vi "WCA_GET_CLNA.vi"(0 "Cartridge Band":u32=10, 1 "Slave Node in":cluster{"Address":i16, "Serial Number":i8[]}={"Address"=19, "Serial Number"=[16, 71, 55, 76, 1, 8, 0, -15]} {"Serial Number" format="%.0x"; "Address" format="%.0x"}, 2 "ObjHandle in":u32, 5 "POL":u32, 7 "sb":u32=1, 9 "avg":u32=1, 11 "error in (no error)":errorcluster) -> (4 "ObjHandle out":u32=92930112, 8 "CLNA_monitor":T1 {"Pol0 LNA1 S3 Gate V [V]" format="%.2f"; "Pol0 LNA1 S3 Drain C [mA]" format="%.2f"; "Pol0 LNA1 S3 Drain V [V]" format="%.2f"; "Pol0 LNA1 S2 Gate V [V]" format="%.2f"; "Pol0 LNA1 S2 Drain C [mA]" format="%.2f"; "Pol0 LNA1 S2 Drain V [V]" format="%.2f"; "Pol0 LNA1 S1 Gate V [V]" format="%.2f"; "Pol0 LNA1 S1 Drain C [mA]" format="%.2f"; "Pol0 LNA1 S1 Drain V [V]" format="%.2f"}, 15 "error out":errorcluster)   [LabVIEW 2017]
uses:
  WCA_Global.vi
  <vilib>/express/express arith-compare/Formula/XNode/ExpressFormulaBlockNode.xnode
panel:
  # "CLNA State."
  # "Vd [V]"
  # "Id [mA]"
  # "Vg [V]"
  # "Stage 1"
  # "Stage 2"
  # "Stage 3"
  # "Node Address"
  # "Serial Number"
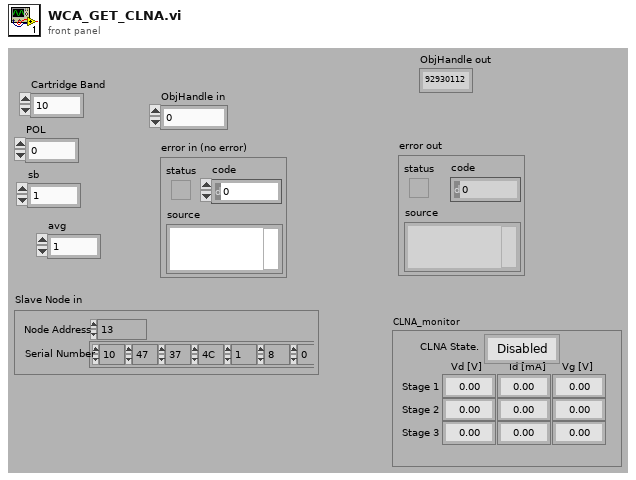
[diagram p1: front panel]
types:
  T1 = cluster{"Pol0 LNA1 S1 Drain V [V]":sgl, "Pol0 LNA1 S1 Drain C [mA]":sgl, "Pol0 LNA1 S1 Gate V [V]":sgl, "Pol0 LNA1 S2 Drain V [V]":sgl, "Pol0 LNA1 S2 Drain C [mA]":sgl, "Pol0 LNA1 S2 Gate V [V]":sgl, "Pol0 LNA1 S3 Drain V [V]":sgl, "Pol0 LNA1 S3 Drain C [mA]":sgl, "Pol0 LNA1 S3 Gate V [V]":sgl, "Pol0 LNA1 State":enum16{"Disabled", "Enabled"}}
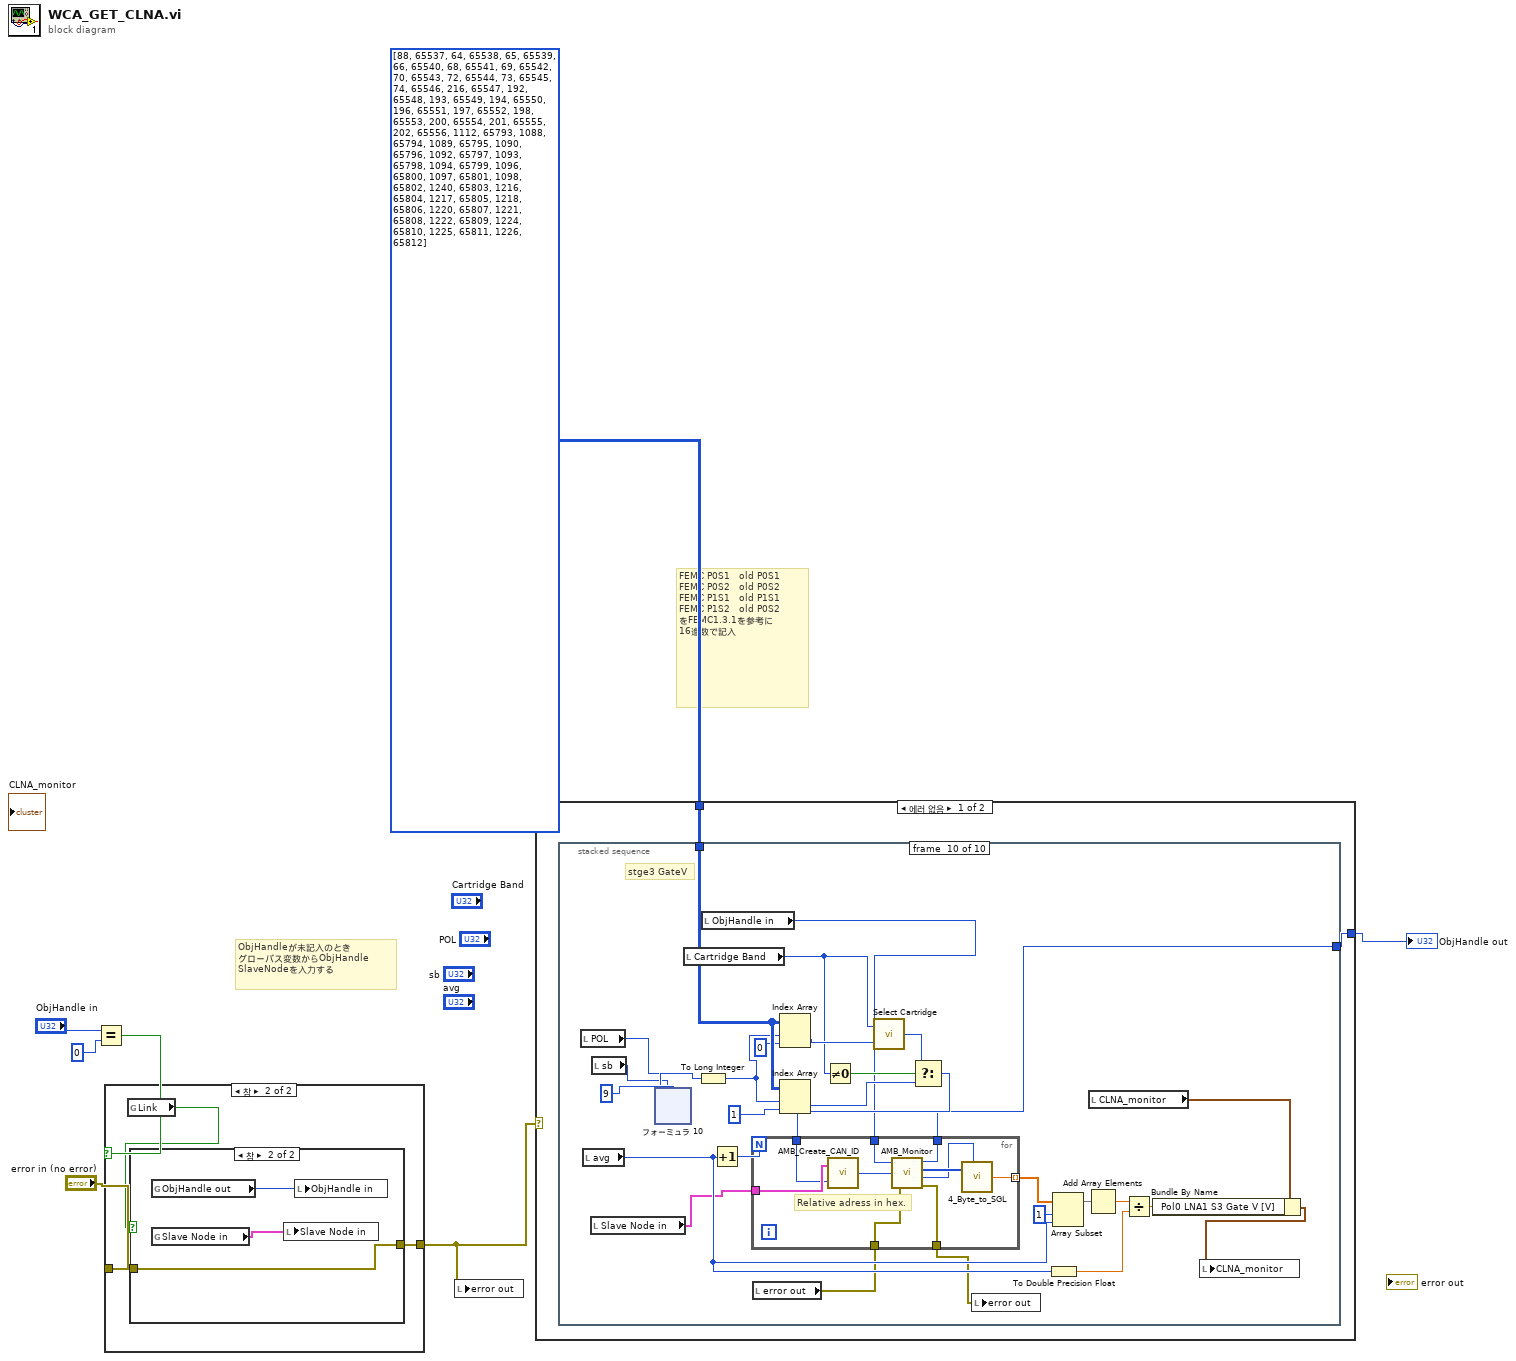
[diagram p0: block diagram]
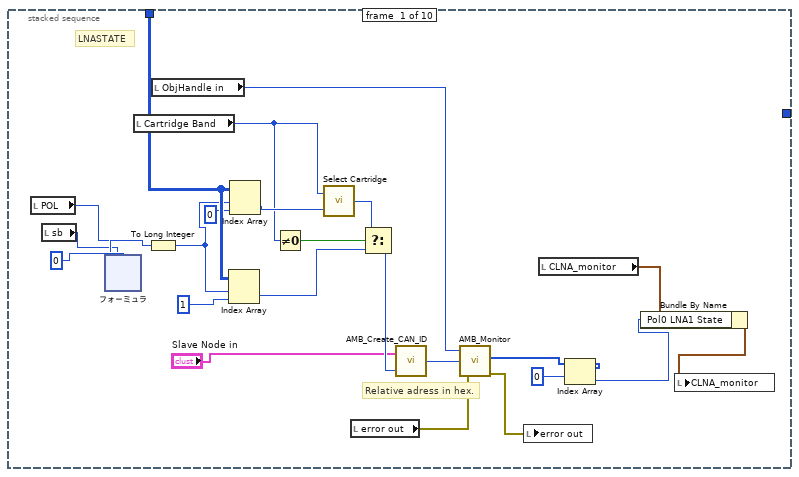
[diagram p2: hidden frame]
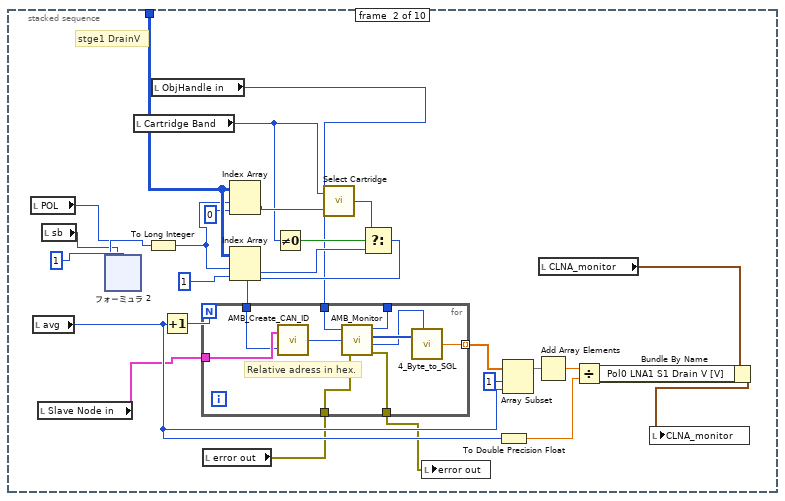
[diagram p3: hidden frame]
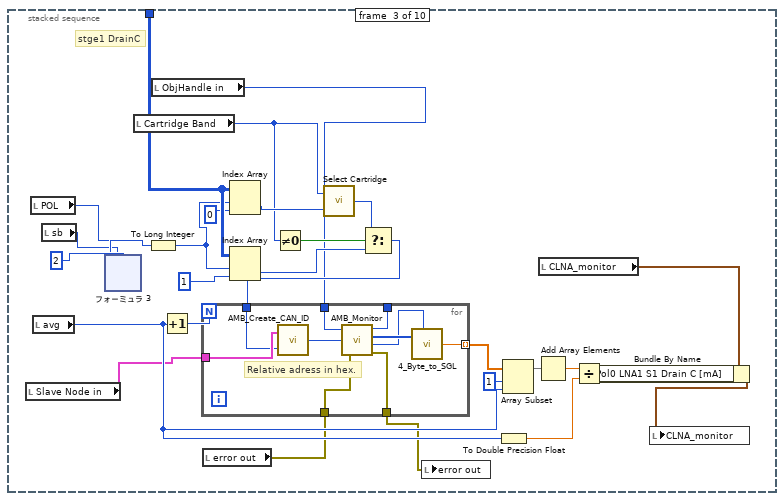
[diagram p4: hidden frame]
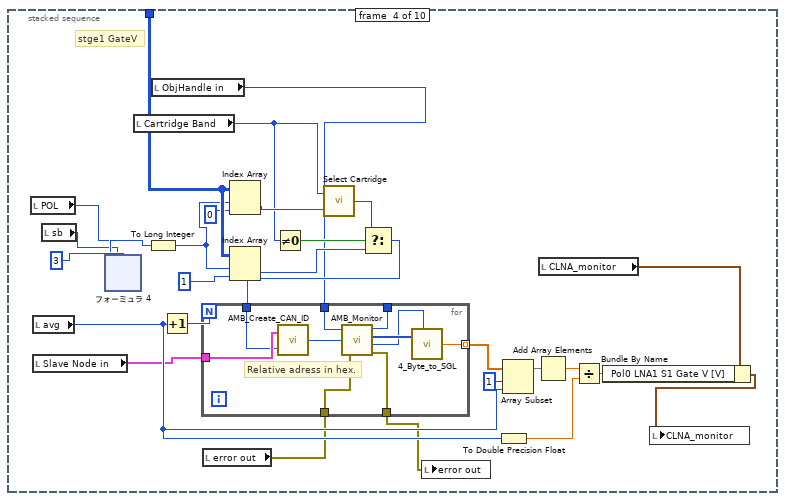
[diagram p5: hidden frame]
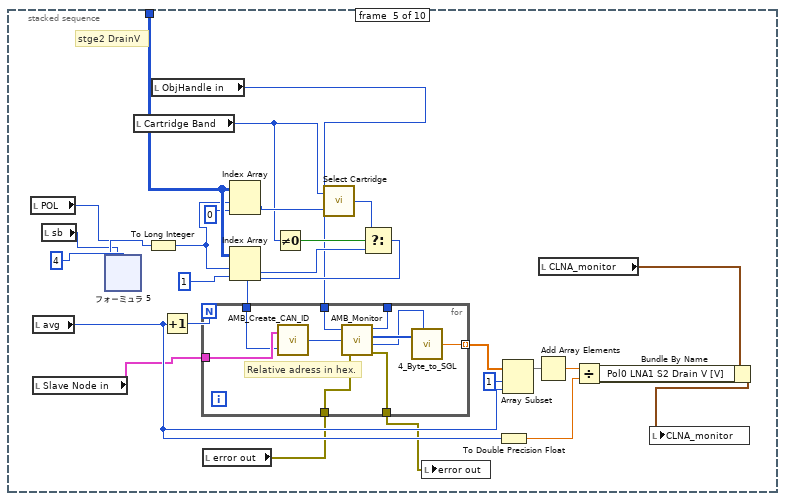
[diagram p6: hidden frame]
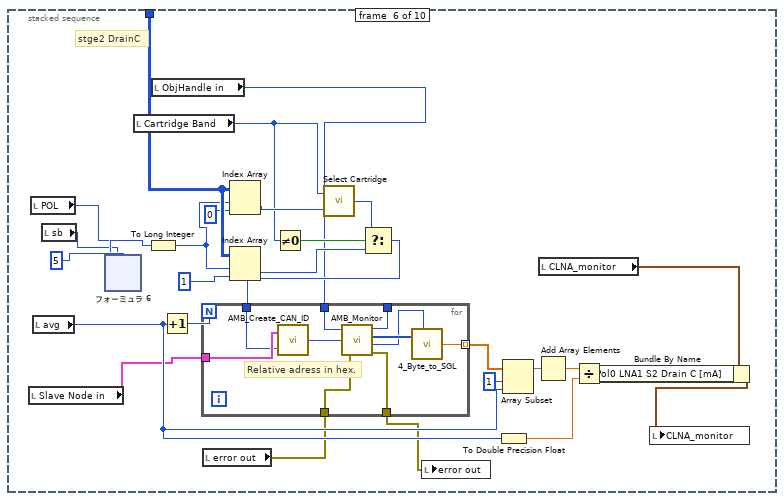
[diagram p7: hidden frame]
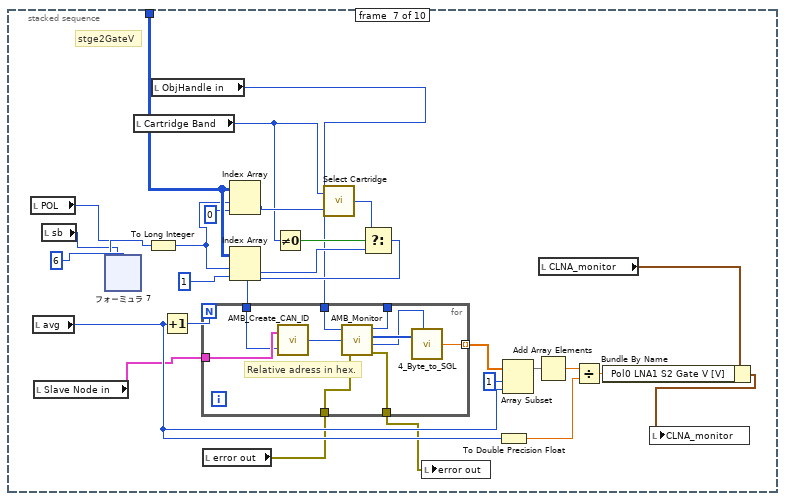
[diagram p8: hidden frame]
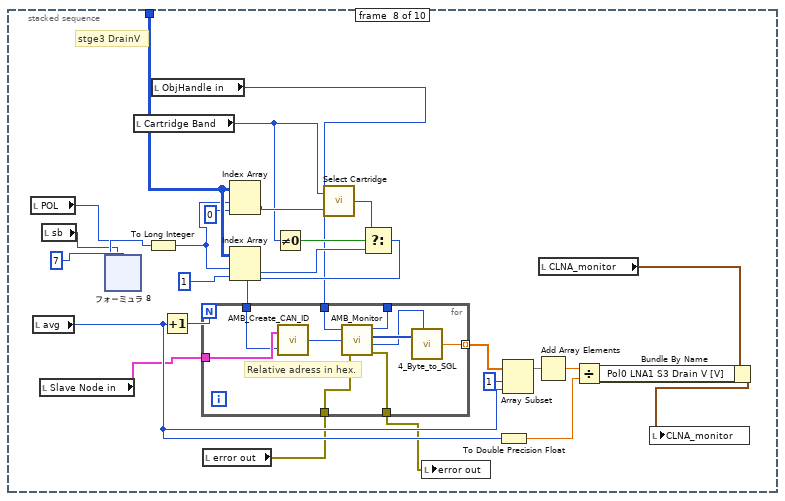
[diagram p9: hidden frame]
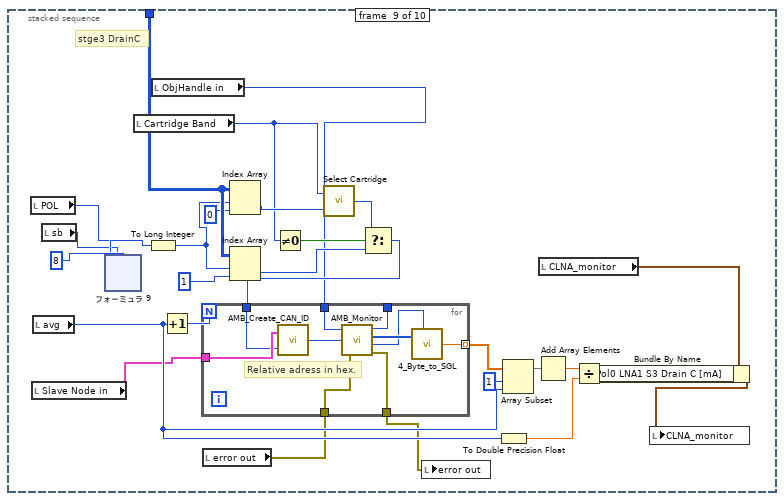
[diagram p10: hidden frame]
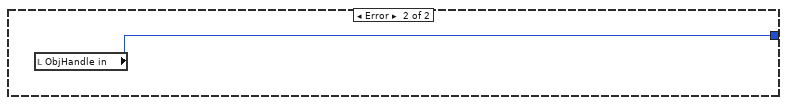
[diagram p11: hidden frame]
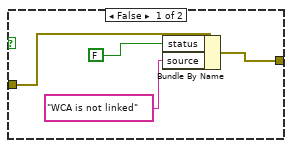
[diagram p13: hidden frame]
diagram:
  # "ObjHandleが未記入のとき\nグローバス変数からObjHandle\nSlaveNodeを入力する"
  # "FEMC P0S1   old P0S1\nFEMC P0S2   old P0S2\nFEMC P1S1   old P1S1\nFEMC P1S2   old P0S2\nをFEMC1.3.1を参考に\n16進数で記入"
  n1 = Equal?(x="ObjHandle in", y=0) -> (x = y?=w5:bool)
  n2 = case shown="참" w5 {
    tunnel: "error in (no error)" -> [w8 w11]
    tunnel: [w8 w10] -> w2
    frame False {
    }
    frame True {
      n3 = global read "WCA_Global.vi" "Link"() -> (w9:bool)
      n4 = case shown="참" w9 {
        tunnel: w11 -> [w15 w16]
        tunnel: [w12 w16] -> w10
        frame False {
          n5 = Bundle By Name(cluster=w15, "status"=FALSE, "source"="WCA is not linked") -> (w12:errorcluster)
        }
        frame True {
          n6 = global read "WCA_Global.vi" "ObjHandle out"() -> (w18:u32)
          n7 = global read "WCA_Global.vi" "Slave Node in"() -> (w17:cluster{"Address":i16, "Serial Number":i8[]})
          n8 = local write "Slave Node in"(w17) -> ()
          n9 = local write "ObjHandle in"(w18) -> ()
        }
      }
    }
  }
  n10 = local write "error out"(w2) -> ()
  n11 = case shown="에러 없음" w2 {
    tunnel: [w19 w508] -> w1
    tunnel: i32[][] [[88, 65537], [64, 65538], [65, 65539], [66, 65540], [68, 65541], [69, 65542], [70, 65543], [72, 65544], [73, 65545], [74, 65546], [216, 65547], [192, 65548], [193, 65549], [194, 65550], [196, 65551], [197, 65552], [198, 65553], [200, 65554], [201, 65555], [202, 65556], [1112, 65793], [1088, 65794], [1089, 65795], [1090, 65796], [1092, 65797], [1093, 65798], [1094, 65799], [1096, 65800], [1097, 65801], [1098, 65802], [1240, 65803], [1216, 65804], [1217, 65805], [1218, 65806], [1220, 65807], [1221, 65808], [1222, 65809], [1224, 65810], [1225, 65811], [1226, 65812]] -> [w20 _]
    frame No Error {
      n12 = stacked-sequence {
        tunnel: w20 -> [w44 w84 w134 w184 w234 w284 w334 w384 w434 w485]
        tunnel: [_ _ _ _ _ _ _ _ _ w457] -> w19
        frame #0 {
          # "Relative adress in hex."
          # "LNASTATE"
          n13 = local read "POL"() -> (w22:u32)
          n14 = local read "sb"() -> (w21:u32)
          n15 = xnode "フォーミュラ"("Pol"=w22, "sb"=w21, "n"=0) -> ("結果"=w33:u32)  [unwired: 1 in, 1 out]
          n16 = local read "Cartridge Band"() -> (w23:u32)
          n17 = To Long Integer(number=w33) -> (32bit integer=w32:i32)
          n18 = local read "ObjHandle in"() -> (w39:u32)
          n19 = Index Array(array=w44, index (row)=w32, index (col)=1) -> (element=w38:i32)
          n20 = Index Array(array=w44, index (row)=w32, index (col)=0) -> (element=w37:i32)
          n21 = Not Equal To 0?(x=w23) -> (x != 0?=w41:bool)
          n22 = call "Select Cartridge.vi"("Relative Address in"=w37, "Cartridge band"=w23) -> ("Relative Address out"=w42:u32)
          n23 = local read "error out"() -> (w25:errorcluster)
          n24 = Select(t=w42, s=w41, f=w38) -> (s? t:f=w43:u32)
          n25 = call "AMB_Create_CAN_ID.vi"("Relative Address in"=w43, "Slave Node in"="Slave Node in") -> ("CAN ID out"=w31:u32)
          n26 = call "AMB_Monitor.vi"("ObjHandle in"=w39, "CAN ID in"=w31, "error in"=w25) -> ("Data Array out"=w30:u8[], "error out"=w24:errorcluster)  [unwired: 2 out]
          n27 = local write "error out"(w24) -> ()
          n28 = local read "CLNA_monitor"() -> (w28:T1)
          n29 = Index Array(array=w30, index=0) -> (element=w27:u8)
          n30 = Bundle By Name(cluster=w28, "Pol0 LNA1 State"=w27) -> (w26:T1)
          n31 = local write "CLNA_monitor"(w26) -> ()
        }
        frame #1 {
          # "stge1 DrainV"
          n32 = local read "POL"() -> (w71:u32)
          n33 = local read "avg"() -> (w63:u32)
          n34 = local read "Slave Node in"() -> (w57:cluster{"Address":i16, "Serial Number":i8[]})
          n35 = local read "sb"() -> (w70:u32)
          n36 = xnode "フォーミュラ 2"("Pol"=w71, "sb"=w70, "n"=1) -> ("結果"=w76:u32)  [unwired: 1 in, 1 out]
          n37 = local read "Cartridge Band"() -> (w72:u32)
          n38 = To Long Integer(number=w76) -> (32bit integer=w75:i32)
          n39 = local read "ObjHandle in"() -> (w61:u32)
          n40 = Increment(x=w63) -> (x+1=w65:u32)
          n41 = local read "error out"() -> (w59:errorcluster)
          n42 = Index Array(array=w84, index (row)=w75, index (col)=0) -> (element=w80:i32)
          n43 = Index Array(array=w84, index (row)=w75, index (col)=1) -> (element=w81:i32)
          n44 = Not Equal To 0?(x=w72) -> (x != 0?=w82:bool)
          n45 = call "Select Cartridge.vi"("Relative Address in"=w80, "Cartridge band"=w72) -> ("Relative Address out"=w83:u32)
          n46 = Select(t=w83, s=w82, f=w81) -> (s? t:f=w62:u32)
          n47 = for {
            N: w65 -> [_]
            tunnel: [w105] -> _
            tunnel: [w104] -> w58
            tunnel: [w102] -> w66 mode=indexing
            tunnel: w57 -> [w100]
            tunnel: w62 -> [w99]
            tunnel: w61 -> [w98]
            tunnel: w59 -> [w97]
            # "Relative adress in hex."
            n48 = call "AMB_Create_CAN_ID.vi"("Relative Address in"=w99, "Slave Node in"=w100) -> ("CAN ID out"=w106:u32)
            n49 = call "AMB_Monitor.vi"("ObjHandle in"=w98, "CAN ID in"=w106, "error in"=w97) -> ("ObjHandle out"=w105:u32, "Data Array out"=w103:u8[], "Data Length out"=w101:u8, "error out"=w104:errorcluster)
            n50 = call "4_Byte_to_SGL.vi"("Array of 4 bytes"=w103, "number of valid bytes"=w101) -> ("Number"=w102:sgl)  [unwired: 1 out]
          }
          n51 = local write "error out"(w58) -> ()
          n52 = To Double Precision Float(number=w63) -> (double precision float=w64:dbl)
          n53 = Array Subset(array=w66, index=1, length=w63) -> (w68:sgl[])
          n54 = Add Array Elements(numeric array=w68) -> (sum=w69:sgl)
          n55 = local read "CLNA_monitor"() -> (w74:T1)
          n56 = Divide(x=w69, y=w64) -> (x/y=w60:dbl)
          n57 = Bundle By Name(cluster=w74, "Pol0 LNA1 S1 Drain V [V]"=w60) -> (w73:T1)
          n58 = local write "CLNA_monitor"(w73) -> ()
        }
        frame #2 {
          # "stge1 DrainC"
          n59 = local read "Slave Node in"() -> (w107:cluster{"Address":i16, "Serial Number":i8[]})
          n60 = local read "POL"() -> (w121:u32)
          n61 = local read "avg"() -> (w113:u32)
          n62 = local read "sb"() -> (w120:u32)
          n63 = xnode "フォーミュラ 3"("Pol"=w121, "sb"=w120, "n"=2) -> ("結果"=w126:u32)  [unwired: 1 in, 1 out]
          n64 = local read "Cartridge Band"() -> (w122:u32)
          n65 = To Long Integer(number=w126) -> (32bit integer=w125:i32)
          n66 = local read "ObjHandle in"() -> (w111:u32)
          n67 = Increment(x=w113) -> (x+1=w115:u32)
          n68 = local read "error out"() -> (w109:errorcluster)
          n69 = Index Array(array=w134, index (row)=w125, index (col)=0) -> (element=w130:i32)
          n70 = Index Array(array=w134, index (row)=w125, index (col)=1) -> (element=w131:i32)
          n71 = Not Equal To 0?(x=w122) -> (x != 0?=w132:bool)
          n72 = call "Select Cartridge.vi"("Relative Address in"=w130, "Cartridge band"=w122) -> ("Relative Address out"=w133:u32)
          n73 = Select(t=w133, s=w132, f=w131) -> (s? t:f=w112:u32)
          n74 = for {
            N: w115 -> [_]
            tunnel: [w155] -> _
            tunnel: [w154] -> w108
            tunnel: [w152] -> w116 mode=indexing
            tunnel: w107 -> [w150]
            tunnel: w112 -> [w149]
            tunnel: w111 -> [w148]
            tunnel: w109 -> [w147]
            # "Relative adress in hex."
            n75 = call "AMB_Create_CAN_ID.vi"("Relative Address in"=w149, "Slave Node in"=w150) -> ("CAN ID out"=w156:u32)
            n76 = call "AMB_Monitor.vi"("ObjHandle in"=w148, "CAN ID in"=w156, "error in"=w147) -> ("ObjHandle out"=w155:u32, "Data Array out"=w153:u8[], "Data Length out"=w151:u8, "error out"=w154:errorcluster)
            n77 = call "4_Byte_to_SGL.vi"("Array of 4 bytes"=w153, "number of valid bytes"=w151) -> ("Number"=w152:sgl)  [unwired: 1 out]
          }
          n78 = local write "error out"(w108) -> ()
          n79 = To Double Precision Float(number=w113) -> (double precision float=w114:dbl)
          n80 = Array Subset(array=w116, index=1, length=w113) -> (w118:sgl[])
          n81 = Add Array Elements(numeric array=w118) -> (sum=w119:sgl)
          n82 = local read "CLNA_monitor"() -> (w124:T1)
          n83 = Divide(x=w119, y=w114) -> (x/y=w110:dbl)
          n84 = Bundle By Name(cluster=w124, "Pol0 LNA1 S1 Drain C [mA]"=w110) -> (w123:T1)
          n85 = local write "CLNA_monitor"(w123) -> ()
        }
        frame #3 {
          # "stge1 GateV"
          n86 = local read "POL"() -> (w171:u32)
          n87 = local read "avg"() -> (w163:u32)
          n88 = local read "Slave Node in"() -> (w157:cluster{"Address":i16, "Serial Number":i8[]})
          n89 = local read "sb"() -> (w170:u32)
          n90 = xnode "フォーミュラ 4"("Pol"=w171, "sb"=w170, "n"=3) -> ("結果"=w176:u32)  [unwired: 1 in, 1 out]
          n91 = local read "Cartridge Band"() -> (w172:u32)
          n92 = To Long Integer(number=w176) -> (32bit integer=w175:i32)
          n93 = local read "ObjHandle in"() -> (w161:u32)
          n94 = Increment(x=w163) -> (x+1=w165:u32)
          n95 = local read "error out"() -> (w159:errorcluster)
          n96 = Index Array(array=w184, index (row)=w175, index (col)=0) -> (element=w180:i32)
          n97 = Index Array(array=w184, index (row)=w175, index (col)=1) -> (element=w181:i32)
          n98 = Not Equal To 0?(x=w172) -> (x != 0?=w182:bool)
          n99 = call "Select Cartridge.vi"("Relative Address in"=w180, "Cartridge band"=w172) -> ("Relative Address out"=w183:u32)
          n100 = Select(t=w183, s=w182, f=w181) -> (s? t:f=w162:u32)
          n101 = for {
            N: w165 -> [_]
            tunnel: [w205] -> _
            tunnel: [w204] -> w158
            tunnel: [w202] -> w166 mode=indexing
            tunnel: w157 -> [w200]
            tunnel: w162 -> [w199]
            tunnel: w161 -> [w198]
            tunnel: w159 -> [w197]
            # "Relative adress in hex."
            n102 = call "AMB_Create_CAN_ID.vi"("Relative Address in"=w199, "Slave Node in"=w200) -> ("CAN ID out"=w206:u32)
            n103 = call "AMB_Monitor.vi"("ObjHandle in"=w198, "CAN ID in"=w206, "error in"=w197) -> ("ObjHandle out"=w205:u32, "Data Array out"=w203:u8[], "Data Length out"=w201:u8, "error out"=w204:errorcluster)
            n104 = call "4_Byte_to_SGL.vi"("Array of 4 bytes"=w203, "number of valid bytes"=w201) -> ("Number"=w202:sgl)  [unwired: 1 out]
          }
          n105 = local write "error out"(w158) -> ()
          n106 = To Double Precision Float(number=w163) -> (double precision float=w164:dbl)
          n107 = Array Subset(array=w166, index=1, length=w163) -> (w168:sgl[])
          n108 = Add Array Elements(numeric array=w168) -> (sum=w169:sgl)
          n109 = local read "CLNA_monitor"() -> (w174:T1)
          n110 = Divide(x=w169, y=w164) -> (x/y=w160:dbl)
          n111 = Bundle By Name(cluster=w174, "Pol0 LNA1 S1 Gate V [V]"=w160) -> (w173:T1)
          n112 = local write "CLNA_monitor"(w173) -> ()
        }
        frame #4 {
          # "stge2 DrainV"
          n113 = local read "POL"() -> (w221:u32)
          n114 = local read "avg"() -> (w213:u32)
          n115 = local read "Slave Node in"() -> (w207:cluster{"Address":i16, "Serial Number":i8[]})
          n116 = local read "sb"() -> (w220:u32)
          n117 = xnode "フォーミュラ 5"("Pol"=w221, "sb"=w220, "n"=4) -> ("結果"=w226:u32)  [unwired: 1 in, 1 out]
          n118 = local read "Cartridge Band"() -> (w222:u32)
          n119 = To Long Integer(number=w226) -> (32bit integer=w225:i32)
          n120 = local read "ObjHandle in"() -> (w211:u32)
          n121 = Increment(x=w213) -> (x+1=w215:u32)
          n122 = local read "error out"() -> (w209:errorcluster)
          n123 = Index Array(array=w234, index (row)=w225, index (col)=0) -> (element=w230:i32)
          n124 = Index Array(array=w234, index (row)=w225, index (col)=1) -> (element=w231:i32)
          n125 = Not Equal To 0?(x=w222) -> (x != 0?=w232:bool)
          n126 = call "Select Cartridge.vi"("Relative Address in"=w230, "Cartridge band"=w222) -> ("Relative Address out"=w233:u32)
          n127 = Select(t=w233, s=w232, f=w231) -> (s? t:f=w212:u32)
          n128 = for {
            N: w215 -> [_]
            tunnel: [w255] -> _
            tunnel: [w254] -> w208
            tunnel: [w252] -> w216 mode=indexing
            tunnel: w207 -> [w250]
            tunnel: w212 -> [w249]
            tunnel: w211 -> [w248]
            tunnel: w209 -> [w247]
            # "Relative adress in hex."
            n129 = call "AMB_Create_CAN_ID.vi"("Relative Address in"=w249, "Slave Node in"=w250) -> ("CAN ID out"=w256:u32)
            n130 = call "AMB_Monitor.vi"("ObjHandle in"=w248, "CAN ID in"=w256, "error in"=w247) -> ("ObjHandle out"=w255:u32, "Data Array out"=w253:u8[], "Data Length out"=w251:u8, "error out"=w254:errorcluster)
            n131 = call "4_Byte_to_SGL.vi"("Array of 4 bytes"=w253, "number of valid bytes"=w251) -> ("Number"=w252:sgl)  [unwired: 1 out]
          }
          n132 = local write "error out"(w208) -> ()
          n133 = To Double Precision Float(number=w213) -> (double precision float=w214:dbl)
          n134 = Array Subset(array=w216, index=1, length=w213) -> (w218:sgl[])
          n135 = Add Array Elements(numeric array=w218) -> (sum=w219:sgl)
          n136 = local read "CLNA_monitor"() -> (w224:T1)
          n137 = Divide(x=w219, y=w214) -> (x/y=w210:dbl)
          n138 = Bundle By Name(cluster=w224, "Pol0 LNA1 S2 Drain V [V]"=w210) -> (w223:T1)
          n139 = local write "CLNA_monitor"(w223) -> ()
        }
        frame #5 {
          # "stge2 DrainC"
          n140 = local read "Slave Node in"() -> (w257:cluster{"Address":i16, "Serial Number":i8[]})
          n141 = local read "POL"() -> (w271:u32)
          n142 = local read "avg"() -> (w263:u32)
          n143 = local read "sb"() -> (w270:u32)
          n144 = xnode "フォーミュラ 6"("Pol"=w271, "sb"=w270, "n"=5) -> ("結果"=w276:u32)  [unwired: 1 in, 1 out]
          n145 = local read "Cartridge Band"() -> (w272:u32)
          n146 = To Long Integer(number=w276) -> (32bit integer=w275:i32)
          n147 = local read "ObjHandle in"() -> (w261:u32)
          n148 = Increment(x=w263) -> (x+1=w265:u32)
          n149 = local read "error out"() -> (w259:errorcluster)
          n150 = Index Array(array=w284, index (row)=w275, index (col)=0) -> (element=w280:i32)
          n151 = Index Array(array=w284, index (row)=w275, index (col)=1) -> (element=w281:i32)
          n152 = Not Equal To 0?(x=w272) -> (x != 0?=w282:bool)
          n153 = call "Select Cartridge.vi"("Relative Address in"=w280, "Cartridge band"=w272) -> ("Relative Address out"=w283:u32)
          n154 = Select(t=w283, s=w282, f=w281) -> (s? t:f=w262:u32)
          n155 = for {
            N: w265 -> [_]
            tunnel: [w305] -> _
            tunnel: [w304] -> w258
            tunnel: [w302] -> w266 mode=indexing
            tunnel: w257 -> [w300]
            tunnel: w262 -> [w299]
            tunnel: w261 -> [w298]
            tunnel: w259 -> [w297]
            # "Relative adress in hex."
            n156 = call "AMB_Create_CAN_ID.vi"("Relative Address in"=w299, "Slave Node in"=w300) -> ("CAN ID out"=w306:u32)
            n157 = call "AMB_Monitor.vi"("ObjHandle in"=w298, "CAN ID in"=w306, "error in"=w297) -> ("ObjHandle out"=w305:u32, "Data Array out"=w303:u8[], "Data Length out"=w301:u8, "error out"=w304:errorcluster)
            n158 = call "4_Byte_to_SGL.vi"("Array of 4 bytes"=w303, "number of valid bytes"=w301) -> ("Number"=w302:sgl)  [unwired: 1 out]
          }
          n159 = local write "error out"(w258) -> ()
          n160 = To Double Precision Float(number=w263) -> (double precision float=w264:dbl)
          n161 = Array Subset(array=w266, index=1, length=w263) -> (w268:sgl[])
          n162 = Add Array Elements(numeric array=w268) -> (sum=w269:sgl)
          n163 = local read "CLNA_monitor"() -> (w274:T1)
          n164 = Divide(x=w269, y=w264) -> (x/y=w260:dbl)
          n165 = Bundle By Name(cluster=w274, "Pol0 LNA1 S2 Drain C [mA]"=w260) -> (w273:T1)
          n166 = local write "CLNA_monitor"(w273) -> ()
        }
        frame #6 {
          # "stge2GateV"
          n167 = local read "POL"() -> (w321:u32)
          n168 = local read "avg"() -> (w313:u32)
          n169 = local read "Slave Node in"() -> (w307:cluster{"Address":i16, "Serial Number":i8[]})
          n170 = local read "sb"() -> (w320:u32)
          n171 = xnode "フォーミュラ 7"("Pol"=w321, "sb"=w320, "n"=6) -> ("結果"=w326:u32)  [unwired: 1 in, 1 out]
          n172 = local read "Cartridge Band"() -> (w322:u32)
          n173 = To Long Integer(number=w326) -> (32bit integer=w325:i32)
          n174 = local read "ObjHandle in"() -> (w311:u32)
          n175 = Increment(x=w313) -> (x+1=w315:u32)
          n176 = local read "error out"() -> (w309:errorcluster)
          n177 = Index Array(array=w334, index (row)=w325, index (col)=0) -> (element=w330:i32)
          n178 = Index Array(array=w334, index (row)=w325, index (col)=1) -> (element=w331:i32)
          n179 = Not Equal To 0?(x=w322) -> (x != 0?=w332:bool)
          n180 = call "Select Cartridge.vi"("Relative Address in"=w330, "Cartridge band"=w322) -> ("Relative Address out"=w333:u32)
          n181 = Select(t=w333, s=w332, f=w331) -> (s? t:f=w312:u32)
          n182 = for {
            N: w315 -> [_]
            tunnel: [w355] -> _
            tunnel: [w354] -> w308
            tunnel: [w352] -> w316 mode=indexing
            tunnel: w307 -> [w350]
            tunnel: w312 -> [w349]
            tunnel: w311 -> [w348]
            tunnel: w309 -> [w347]
            # "Relative adress in hex."
            n183 = call "AMB_Create_CAN_ID.vi"("Relative Address in"=w349, "Slave Node in"=w350) -> ("CAN ID out"=w356:u32)
            n184 = call "AMB_Monitor.vi"("ObjHandle in"=w348, "CAN ID in"=w356, "error in"=w347) -> ("ObjHandle out"=w355:u32, "Data Array out"=w353:u8[], "Data Length out"=w351:u8, "error out"=w354:errorcluster)
            n185 = call "4_Byte_to_SGL.vi"("Array of 4 bytes"=w353, "number of valid bytes"=w351) -> ("Number"=w352:sgl)  [unwired: 1 out]
          }
          n186 = local write "error out"(w308) -> ()
          n187 = To Double Precision Float(number=w313) -> (double precision float=w314:dbl)
          n188 = Array Subset(array=w316, index=1, length=w313) -> (w318:sgl[])
          n189 = Add Array Elements(numeric array=w318) -> (sum=w319:sgl)
          n190 = local read "CLNA_monitor"() -> (w324:T1)
          n191 = Divide(x=w319, y=w314) -> (x/y=w310:dbl)
          n192 = Bundle By Name(cluster=w324, "Pol0 LNA1 S2 Gate V [V]"=w310) -> (w323:T1)
          n193 = local write "CLNA_monitor"(w323) -> ()
        }
        frame #7 {
          # "stge3 DrainV"
          n194 = local read "POL"() -> (w371:u32)
          n195 = local read "avg"() -> (w363:u32)
          n196 = local read "Slave Node in"() -> (w357:cluster{"Address":i16, "Serial Number":i8[]})
          n197 = local read "sb"() -> (w370:u32)
          n198 = xnode "フォーミュラ 8"("Pol"=w371, "sb"=w370, "n"=7) -> ("結果"=w376:u32)  [unwired: 1 in, 1 out]
          n199 = local read "Cartridge Band"() -> (w372:u32)
          n200 = To Long Integer(number=w376) -> (32bit integer=w375:i32)
          n201 = local read "ObjHandle in"() -> (w361:u32)
          n202 = Increment(x=w363) -> (x+1=w365:u32)
          n203 = local read "error out"() -> (w359:errorcluster)
          n204 = Index Array(array=w384, index (row)=w375, index (col)=0) -> (element=w380:i32)
          n205 = Index Array(array=w384, index (row)=w375, index (col)=1) -> (element=w381:i32)
          n206 = Not Equal To 0?(x=w372) -> (x != 0?=w382:bool)
          n207 = call "Select Cartridge.vi"("Relative Address in"=w380, "Cartridge band"=w372) -> ("Relative Address out"=w383:u32)
          n208 = Select(t=w383, s=w382, f=w381) -> (s? t:f=w362:u32)
          n209 = for {
            N: w365 -> [_]
            tunnel: [w405] -> _
            tunnel: [w404] -> w358
            tunnel: [w402] -> w366 mode=indexing
            tunnel: w357 -> [w400]
            tunnel: w362 -> [w399]
            tunnel: w361 -> [w398]
            tunnel: w359 -> [w397]
            # "Relative adress in hex."
            n210 = call "AMB_Create_CAN_ID.vi"("Relative Address in"=w399, "Slave Node in"=w400) -> ("CAN ID out"=w406:u32)
            n211 = call "AMB_Monitor.vi"("ObjHandle in"=w398, "CAN ID in"=w406, "error in"=w397) -> ("ObjHandle out"=w405:u32, "Data Array out"=w403:u8[], "Data Length out"=w401:u8, "error out"=w404:errorcluster)
            n212 = call "4_Byte_to_SGL.vi"("Array of 4 bytes"=w403, "number of valid bytes"=w401) -> ("Number"=w402:sgl)  [unwired: 1 out]
          }
          n213 = local write "error out"(w358) -> ()
          n214 = To Double Precision Float(number=w363) -> (double precision float=w364:dbl)
          n215 = Array Subset(array=w366, index=1, length=w363) -> (w368:sgl[])
          n216 = Add Array Elements(numeric array=w368) -> (sum=w369:sgl)
          n217 = local read "CLNA_monitor"() -> (w374:T1)
          n218 = Divide(x=w369, y=w364) -> (x/y=w360:dbl)
          n219 = Bundle By Name(cluster=w374, "Pol0 LNA1 S3 Drain V [V]"=w360) -> (w373:T1)
          n220 = local write "CLNA_monitor"(w373) -> ()
        }
        frame #8 {
          # "stge3 DrainC"
          n221 = local read "POL"() -> (w421:u32)
          n222 = local read "Slave Node in"() -> (w407:cluster{"Address":i16, "Serial Number":i8[]})
          n223 = local read "avg"() -> (w413:u32)
          n224 = local read "sb"() -> (w420:u32)
          n225 = xnode "フォーミュラ 9"("Pol"=w421, "sb"=w420, "n"=8) -> ("結果"=w426:u32)  [unwired: 1 in, 1 out]
          n226 = local read "Cartridge Band"() -> (w422:u32)
          n227 = To Long Integer(number=w426) -> (32bit integer=w425:i32)
          n228 = local read "ObjHandle in"() -> (w411:u32)
          n229 = Increment(x=w413) -> (x+1=w415:u32)
          n230 = local read "error out"() -> (w409:errorcluster)
          n231 = Index Array(array=w434, index (row)=w425, index (col)=0) -> (element=w430:i32)
          n232 = Index Array(array=w434, index (row)=w425, index (col)=1) -> (element=w431:i32)
          n233 = Not Equal To 0?(x=w422) -> (x != 0?=w432:bool)
          n234 = call "Select Cartridge.vi"("Relative Address in"=w430, "Cartridge band"=w422) -> ("Relative Address out"=w433:u32)
          n235 = Select(t=w433, s=w432, f=w431) -> (s? t:f=w412:u32)
          n236 = for {
            N: w415 -> [_]
            tunnel: [w455] -> _
            tunnel: [w454] -> w408
            tunnel: [w452] -> w416 mode=indexing
            tunnel: w407 -> [w450]
            tunnel: w412 -> [w449]
            tunnel: w411 -> [w448]
            tunnel: w409 -> [w447]
            # "Relative adress in hex."
            n237 = call "AMB_Create_CAN_ID.vi"("Relative Address in"=w449, "Slave Node in"=w450) -> ("CAN ID out"=w456:u32)
            n238 = call "AMB_Monitor.vi"("ObjHandle in"=w448, "CAN ID in"=w456, "error in"=w447) -> ("ObjHandle out"=w455:u32, "Data Array out"=w453:u8[], "Data Length out"=w451:u8, "error out"=w454:errorcluster)
            n239 = call "4_Byte_to_SGL.vi"("Array of 4 bytes"=w453, "number of valid bytes"=w451) -> ("Number"=w452:sgl)  [unwired: 1 out]
          }
          n240 = local write "error out"(w408) -> ()
          n241 = To Double Precision Float(number=w413) -> (double precision float=w414:dbl)
          n242 = Array Subset(array=w416, index=1, length=w413) -> (w418:sgl[])
          n243 = Add Array Elements(numeric array=w418) -> (sum=w419:sgl)
          n244 = local read "CLNA_monitor"() -> (w424:T1)
          n245 = Divide(x=w419, y=w414) -> (x/y=w410:dbl)
          n246 = Bundle By Name(cluster=w424, "Pol0 LNA1 S3 Drain C [mA]"=w410) -> (w423:T1)
          n247 = local write "CLNA_monitor"(w423) -> ()
        }
        frame #9 {
          # "stge3 GateV"
          n248 = local read "POL"() -> (w472:u32)
          n249 = local read "avg"() -> (w464:u32)
          n250 = local read "Slave Node in"() -> (w458:cluster{"Address":i16, "Serial Number":i8[]})
          n251 = local read "sb"() -> (w471:u32)
          n252 = xnode "フォーミュラ 10"("Pol"=w472, "sb"=w471, "n"=9) -> ("結果"=w477:u32)  [unwired: 1 in, 1 out]
          n253 = local read "Cartridge Band"() -> (w473:u32)
          n254 = To Long Integer(number=w477) -> (32bit integer=w476:i32)
          n255 = local read "ObjHandle in"() -> (w462:u32)
          n256 = Increment(x=w464) -> (x+1=w466:u32)
          n257 = local read "error out"() -> (w460:errorcluster)
          n258 = Index Array(array=w485, index (row)=w476, index (col)=0) -> (element=w481:i32)
          n259 = Index Array(array=w485, index (row)=w476, index (col)=1) -> (element=w482:i32)
          n260 = Not Equal To 0?(x=w473) -> (x != 0?=w483:bool)
          n261 = call "Select Cartridge.vi"("Relative Address in"=w481, "Cartridge band"=w473) -> ("Relative Address out"=w484:u32)
          n262 = Select(t=w484, s=w483, f=w482) -> (s? t:f=w463:u32)
          n263 = for {
            N: w466 -> [_]
            tunnel: [w506] -> w457
            tunnel: [w505] -> w459
            tunnel: [w503] -> w467 mode=indexing
            tunnel: w458 -> [w501]
            tunnel: w463 -> [w500]
            tunnel: w462 -> [w499]
            tunnel: w460 -> [w498]
            # "Relative adress in hex."
            n264 = call "AMB_Create_CAN_ID.vi"("Relative Address in"=w500, "Slave Node in"=w501) -> ("CAN ID out"=w507:u32)
            n265 = call "AMB_Monitor.vi"("ObjHandle in"=w499, "CAN ID in"=w507, "error in"=w498) -> ("ObjHandle out"=w506:u32, "Data Array out"=w504:u8[], "Data Length out"=w502:u8, "error out"=w505:errorcluster)
            n266 = call "4_Byte_to_SGL.vi"("Array of 4 bytes"=w504, "number of valid bytes"=w502) -> ("Number"=w503:sgl)  [unwired: 1 out]
          }
          n267 = local write "error out"(w459) -> ()
          n268 = To Double Precision Float(number=w464) -> (double precision float=w465:dbl)
          n269 = Array Subset(array=w467, index=1, length=w464) -> (w469:sgl[])
          n270 = Add Array Elements(numeric array=w469) -> (sum=w470:sgl)
          n271 = local read "CLNA_monitor"() -> (w475:T1)
          n272 = Divide(x=w470, y=w465) -> (x/y=w461:dbl)
          n273 = Bundle By Name(cluster=w475, "Pol0 LNA1 S3 Gate V [V]"=w461) -> (w474:T1)
          n274 = local write "CLNA_monitor"(w474) -> ()
        }
      }
    }
    frame Error {
      n275 = local read "ObjHandle in"() -> (w508:u32)
    }
  }
  "ObjHandle out" <- w1
